vi "Compute Calibrated Phasor Array.vi"(6 "Phasor Calibration Data":T7, 7 "Phasor Calculation":T1, 8 "Error In":errorcluster, 9 "Gates Definitions":T4={"First Gate: t1"=0.0, "Gate Width: W"=0.0, "Gate Step: d"=0.0, "# Gates: G"=0.0, "Use Gate Center"=FALSE, "Frames/Image: F"=50, "Gates/Frame: L"=0, "Bits/Frame: q"=0, "Multiplicity: p"=0, "Gate Type"=enum."Square", "Gate Edge s"=4.0, "Gate Top Slope"=4.0, "Reversed Sawtooth?"=FALSE, "Computation"=FALSE, "User-defined Gate"={"X Array"=[], "Y Array"=[]}, "Tolerance"=50.0, "Integration"=enum."Item 0", "# Steps"=50.0, "Type of User-defined Function"=enum."Gate"}, 10 "Decay Definition":T2={"offset: t0"=0.0, "period: T"=0.0, "lifetime: tau"=0.0, "Incident Signal: I"=0.5, "Normalized Decays"=FALSE, "IRF Model"=enum."Dirac", "IRF Parameter 1"=0.0, "Poisson Signal"=FALSE}, 11 "Lifetime Array":ext[](array[numeric])) -> (0 "Error Out":errorcluster, 1 "Calibrated s Array":ext[](array[numeric]), 2 "Calibrated g Array":ext[](array[numeric]), 3 "True Lifetime Array":ext[](array[numeric]), 4 "# Rejected Pairs":i32, 5 "CPU (s)":dbl)   [LabVIEW 2019]
uses:
  Phasor Calibration Data.ctl
  Gate Definitions.ctl
  Gate Type.ctl
  Graphs/XY Graph/XY Plot Data.ctl
  Decay Definiton.ctl
  IRF Model.ctl
  Phasor Calculation Type.ctl
  Phasor_Abort Parallel Computation.vi
  <vilib>/Utility/error.llb/Error Cluster From Error Code.vi
  <vilib>/ErrorRing/Error Ring.xnode
panel:
  out "Uncalibrated Phasors":cxt[](array[numeric])
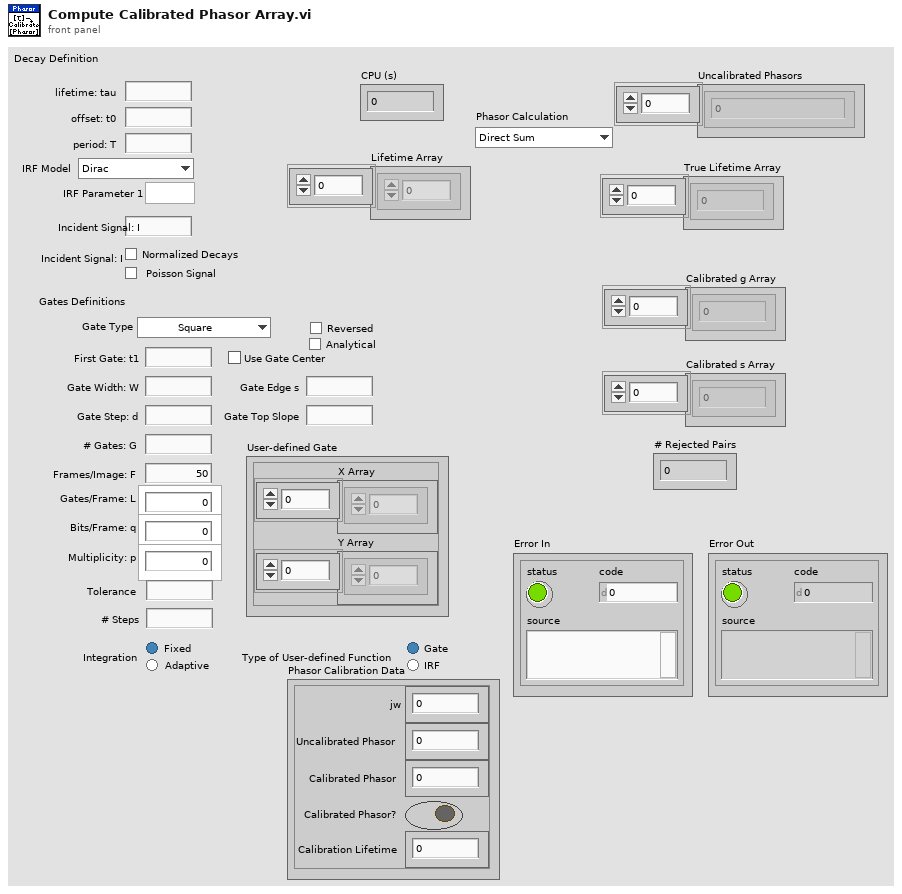
[diagram p1: front panel]
types:
  T1 = typedef "Phasor Calculation Type.ctl" = enum16{"Direct Sum", "Analytical Formula"}
  T2 = typedef "Decay Definiton.ctl" = cluster{"offset: t0":ext, "period: T":ext, "lifetime: tau":ext, "Incident Signal: I":ext, "Normalized Decays":bool, "IRF Model":T3, "IRF Parameter 1":ext, "Poisson Signal":bool}
  T3 = typedef "IRF Model.ctl" = enum16{"Dirac", "Exponential"}
  T4 = typedef "Gate Definitions.ctl" = cluster{"First Gate: t1":ext, "Gate Width: W":ext, "Gate Step: d":ext, "# Gates: G":ext, "Use Gate Center":bool, "Frames/Image: F":i32, "Gates/Frame: L":i32, "Bits/Frame: q":i32, "Multiplicity: p":i32, "Gate Type":T5, "Gate Edge s":ext, "Gate Top Slope":ext, "Reversed Sawtooth?":bool, "Computation":bool, "User-defined Gate":T6, "Tolerance":ext, "Integration":enum32{"Item 0", "Item 1"}, "# Steps":ext, "Type of User-defined Function":enum32{"Gate", "IRF"}}
  T5 = typedef "Gate Type.ctl" = enum16{"Square", "Finite Edge Square", "Finite Edge, Tilted Top Square", "Triangle", "Sawtooth", "User-defined"}
  T6 = typedef "XY Plot Data.ctl" = cluster{"X Array":dbl[], "Y Array":dbl[]}
  T7 = typedef "Phasor Calibration Data.ctl" = cluster{"jw":cxt, "Uncalibrated Phasor":cxt, "Calibrated Phasor":cxt, "Calibrated Phasor?":bool, "Calibration Lifetime":ext}
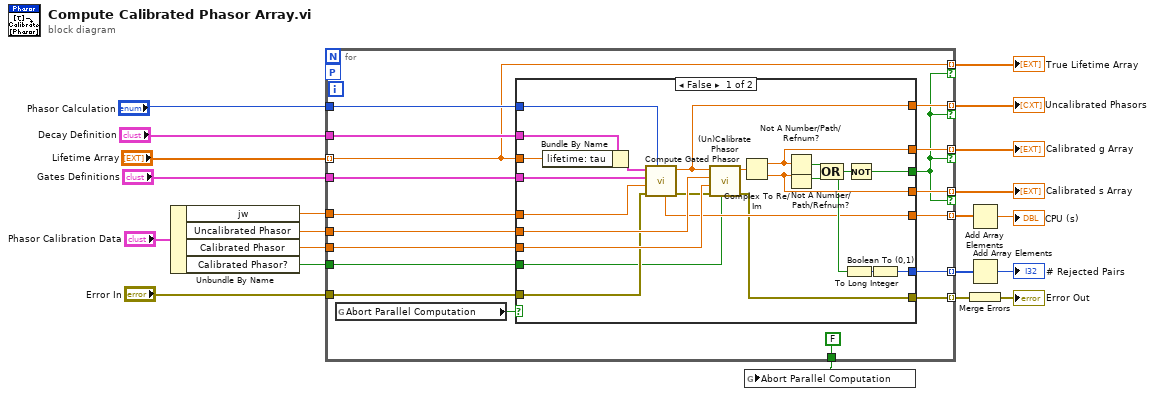
[diagram p0: block diagram]
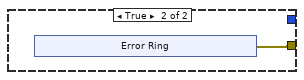
[diagram p2: hidden frame]
diagram:
  n1 = Unbundle By Name("Phasor Calibration Data") -> ("jw"=w18:cxt, "Uncalibrated Phasor"=w19:cxt, "Calibrated Phasor"=w20:cxt, "Calibrated Phasor?"=w21:bool)
  n2 = for {
    tunnel: "Lifetime Array" -> [w22] mode=indexing
    tunnel: w18 -> [w39]
    tunnel: [w32] -> w12 mode=indexing if=w29
    tunnel: [w31] -> w13 mode=indexing if=w29
    tunnel: "Gates Definitions" -> [w38]
    tunnel: "Decay Definition" -> [w37]
    tunnel: w19 -> [w36]
    tunnel: w20 -> [w35]
    tunnel: w21 -> [w26]
    tunnel: "Phasor Calculation" -> [w34]
    tunnel: [w22] -> w8 mode=indexing if=w29
    tunnel: [w30] -> w7 mode=indexing if=w29
    tunnel: "Error In" -> [w33]
    tunnel: [w25] -> w9 mode=indexing
    tunnel: [w28] -> w5 mode=indexing
    tunnel: [w27] -> w3 mode=indexing
    workers-P: _ -> [_]
    tunnel: [FALSE ("Abort Parallel Computation")] -> w1
    n3 = global read "Phasor_Abort Parallel Computation.vi" "Abort Parallel Computation"() -> (w23:bool)
    n4 = case shown="False" w23 {
      tunnel: w39 -> [w61 _]
      tunnel: w38 -> [w60 _]
      tunnel: w37 -> [w59 _]
      tunnel: w36 -> [w57 _]
      tunnel: w35 -> [w56 _]
      tunnel: w34 -> [w55 _]
      tunnel: w33 -> [w54 _]
      tunnel: [w53 _] -> w32
      tunnel: [w52 _] -> w31
      tunnel: w22 -> [w49 _]
      tunnel: [w48 _] -> w30
      tunnel: [w47 _] -> w29
      tunnel: [w44 _] -> w28
      tunnel: [w43 _] -> w27
      tunnel: w26 -> [w42 _]
      tunnel: [w40 w63] -> w25
      frame False {
        n5 = Bundle By Name(cluster=w59, "lifetime: tau"=w49) -> (w62:T2)
        n6 = call "Compute Gated Phasor.vi"("Phasor Calculation Type"=w55, "Error In"=w54, "j 2 pi f"=w61, "Gates Definitions"=w60, "Decay Definition"=w62) -> ("Error Out"=w41:errorcluster, "phasor"=w48:cxt, "CPU (s)"=w43:dbl)  [unwired: 4 in]
        n7 = call "(Un)Calibrate Phasor.vi"("Calibrated Phasor"=w42, "Error In"=w41, "Target Phasor"=w56, "Calibration Phasor"=w57, "Phasor in"=w48) -> ("Error Out"=w40:errorcluster, "Phasor out"=w58:cxt)  [unwired: 5 in]
        n8 = Complex To Re/Im(x + iy=w58) -> (x=w53:ext, y=w52:ext)
        n9 = Not A Number/Path/Refnum?(number/path/refnum=w53) -> (NaN/Path/Refnum?=w51:bool)
        n10 = Not A Number/Path/Refnum?(number/path/refnum=w52) -> (NaN/Path/Refnum?=w50:bool)
        n11 = Compound Arithmetic op=OR(w51, w50) -> (w46:bool)
        n12 = Boolean To (0,1)(Boolean=w46) -> (0, 1=w45:i16)
        n13 = Not(x=w46) -> (.not. x?=w47:bool)
        n14 = To Long Integer(number=w45) -> (32bit integer=w44:i32)
      }
      frame True {
        n15 = xnode "Error Ring"() -> ("error out"=w63:errorcluster)
      }
    }
  }
  "Calibrated s Array" <- w13
  "Calibrated g Array" <- w12
  "True Lifetime Array" <- w8
  "Uncalibrated Phasors" <- w7
  n16 = global write "Phasor_Abort Parallel Computation.vi" "Abort Parallel Computation"(w1) -> ()
  n17 = Add Array Elements(numeric array=w3) -> (sum=→"CPU (s)":dbl)
  n18 = Add Array Elements(numeric array=w5) -> (sum=→"# Rejected Pairs":i32)
  n19 = Merge Errors(w9) -> (→"Error Out":errorcluster)
